vi "U16ToAddress.vi"(1 "Input":i16) -> (0 "Addresses":T1)   [LabVIEW 2018]
uses:
  DataTypes/Addresses.ctl
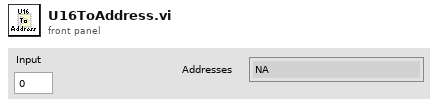
[diagram p1: front panel]
types:
  T1 = typedef "Addresses.ctl" = enum8{"NA", "Accelerometers", "Timestamp", "ChasisTemperature"}
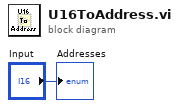
[diagram p0: block diagram]
diagram:
  "Addresses" <- "Input"
